vi "FlatToRichni_measurementlink_sessionmanagement_v1_ReserveAllRegisteredSessionsRequest.vi"(5 "OutputClusterType":T1, 11 "InputCluster":T2) -> (3 "OutputCluster":T1)   [LabVIEW 2024, in "ni.measurementlink.sessionmanagement.v1.api.lvlib"]
uses:
  ni.measurementlink.sessionmanagement.v1.api.lvlib
  ni_measurementlink_sessionmanagement_v1_ReserveAllRegisteredSessionsRequest_Flat.ctl
  ni_measurementlink_sessionmanagement_v1_ReserveAllRegisteredSessionsRequest.ctl
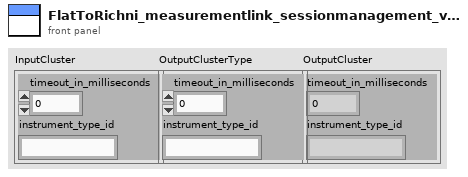
[diagram p1: front panel]
types:
  T1 = typedef "ni.measurementlink.sessionmanagement.v1.api.lvlib/ni_measurementlink_sessionmanagement_v1_ReserveAllRegisteredSessionsRequest.ctl" = cluster{"timeout_in_milliseconds":i32, "instrument_type_id":string}
  T2 = typedef "ni.measurementlink.sessionmanagement.v1.api.lvlib/ni_measurementlink_sessionmanagement_v1_ReserveAllRegisteredSessionsRequest_Flat.ctl" = cluster{"timeout_in_milliseconds":i32, "instrument_type_id":string}
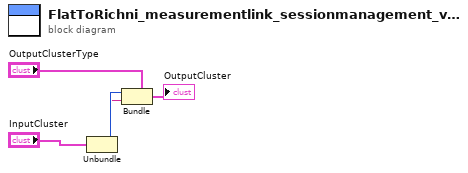
[diagram p0: block diagram]
diagram:
  n1 = Unbundle "Unbundle"("InputCluster") -> ("timeout_in_milliseconds"=w2:i32, "instrument_type_id"=w1:string)
  n2 = Bundle "Bundle"(cluster="OutputClusterType", "timeout_in_milliseconds"=w2, "instrument_type_id"=w1) -> (→"OutputCluster":T1)
